vi "V7310.Variable.Value.Set.vi"(6 "timeout ms (5000)":i32=5000, 8 "error in":errorcluster, 9 "Value":string, 10 "Variable":string, 11 "Connection in":refnum<k5>) -> (0 "error out":errorcluster, 3 "Connection out":refnum<k5>)   [LabVIEW 2016]
uses:
  LowLevel/V7310.Commands.ctl
panel:
  out "Data out":string
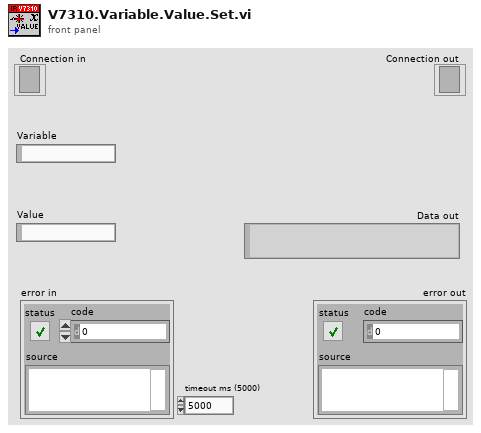
[diagram p1: front panel]
types:
  T1 = typedef "V7310.Commands.ctl" = enum16{"Start", "Stop", "GetStatus", "GetVarNames", "GetJobNames", "SetJob", "GetJob", "SetVars", "GetVars", "SetLayoutPosition", "SetRotation", "GetMessageID", "GetMessages", "ConfirmMessages", "DeleteMessages", "SetRTC", "GetRTC", "SetVarPosition", "SetIntensity", "GetIntensity", "SetStartTriggerDelay", "GetStartTriggerDelay", "SetStopTriggerDelay", "GetStopTriggerDelay", "SetConsecutiveTriggerDelay", "GetConsecutiveTriggerDelay", "SetMarkSpeed", "GetMarkSpeed"}
  T2 = typedef "V7310.ErrorLevels.ctl" = enum16{"OK", "Warning", "Error"}
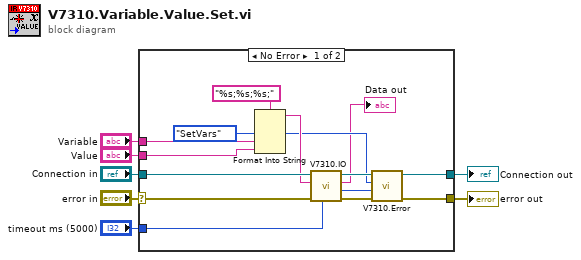
[diagram p0: block diagram]
diagram:
  n1 = case shown="No Error" "error in" {
    selector: "error in" -> [w18 w21]
    tunnel: "Connection in" -> [w19 w22]
    tunnel: [w20 w22] -> w6
    tunnel: "timeout ms (5000)" -> [w17 _]
    tunnel: [w12 w21] -> w3
    tunnel: "Variable" -> [w9 _]
    tunnel: "Value" -> [w8 _]
    frame No Error {
      w11 = V7310.Commands."SetVars" ("Cmd")
      n2 = Format Into String(format string="%s;%s;%s;", w11, w9, w8) -> (resulting string=w15:string)  [unwired: 2 in, 1 out]
      n3 = call "V7310.IO.vi"("timeout ms (5000)"=w17, "error in"=w18, "Data in"=w15, "Connection in"=w19) -> ("error out"=w13:errorcluster, "Error Level"=w14:T2, "Data out"=→"Data out":string, "Connection out"=w20:refnum<k5>)  [unwired: 4 in]
      n4 = call "V7310.Error.vi"("error in"=w13, "Error Level"=w14, "Cmd"=w11) -> ("error out"=w12:errorcluster)  [unwired: 8 in]
    }
    frame Error {
    }
  }
  "Connection out" <- w6
  "error out" <- w3
